vi "Peregrine_write.vi"(0 "Handle in":refnum<visa-resource-name>, 2 "Address":u8, 5 "Key":u32, 7 "Value":i32, 11 "error":errorcluster) -> (4 "Handle out":refnum<visa-resource-name>, 6 "Key response":u32, 8 "Value response":i32, 15 "error out":errorcluster)   [LabVIEW 2019]
panel:
  out "Command":i32
  out "Address response":u8
  # "Inputs"
  # "Response message"
  # "Output"
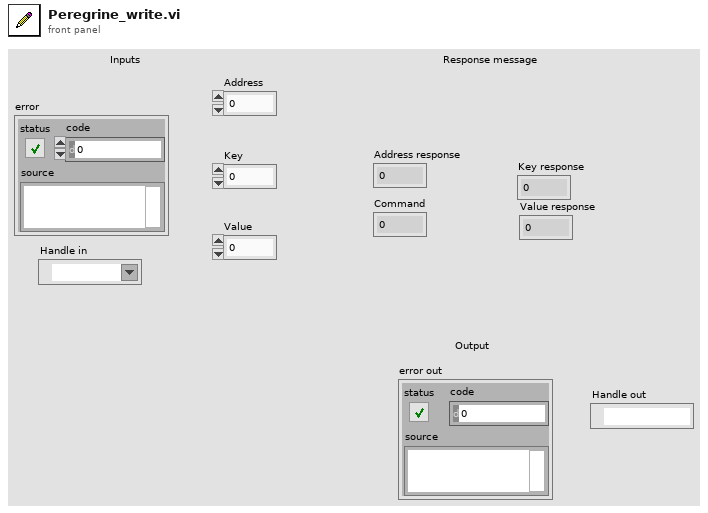
[diagram p1: front panel]
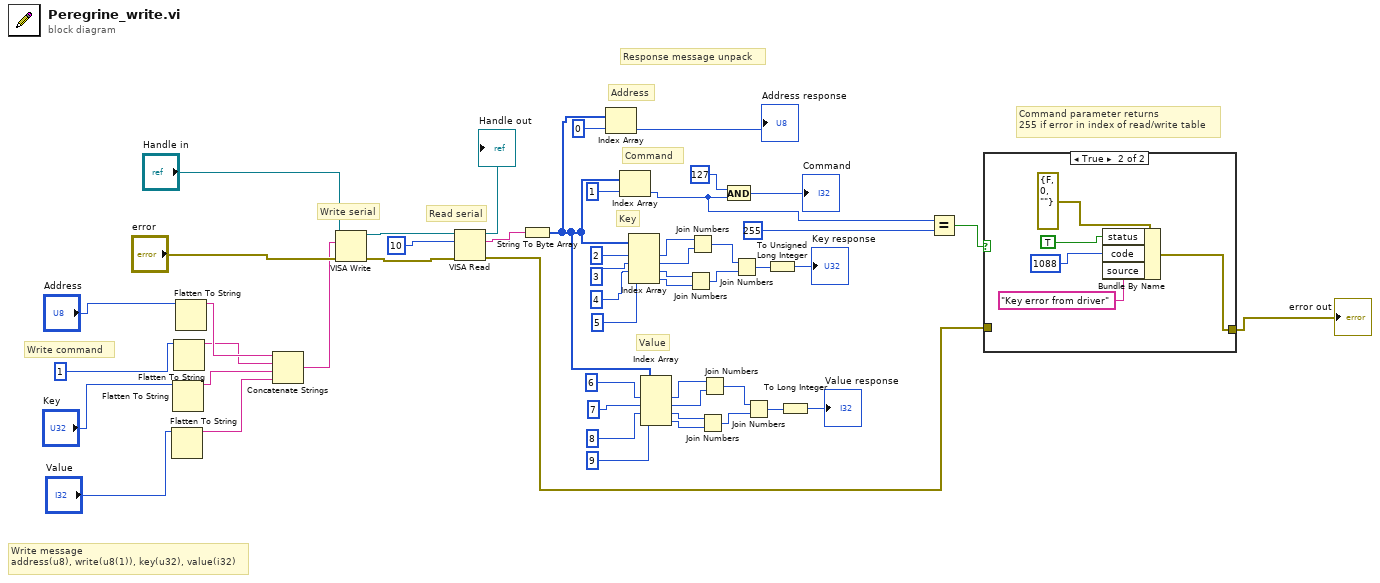
[diagram p0: block diagram]
diagram:
  # "Command parameter returns\n255 if error in index of read/write table"
  # "Value"
  # "Response message unpack"
  # "Write command"
  # "Command"
  # "Address"
  # "Key"
  # "Read serial"
  # "Write serial"
  # "Write message\naddress(u8), write(u8(1)), key(u32), value(i32)"
  n1 = Flatten To String(anything="Value") -> (data string=w24:string)  [unwired: 3 in, 2 out]
  n2 = Flatten To String(anything="Key") -> (data string=w25:string)  [unwired: 3 in, 2 out]
  n3 = Flatten To String(anything=u8 1) -> (data string=w26:string)  [unwired: 3 in, 2 out]
  n4 = Flatten To String(anything="Address") -> (data string=w28:string)  [unwired: 3 in, 2 out]
  n5 = Concatenate Strings(w28, w26, w25, w24) -> (w23:string)
  n6 = VISA Write(VISA resource name="Handle in", write buffer=w23, error in (no error)="error") -> (VISA resource name out=w51:refnum<visa-resource-name>, error out=w30:errorcluster)  [unwired: 1 out]
  n7 = VISA Read(VISA resource name=w51, byte count=10, error in (no error)=w30) -> (VISA resource name out=→"Handle out":refnum<visa-resource-name>, read buffer=w49:string, error out=w3:errorcluster)  [unwired: 1 out]
  n8 = String To Byte Array(string=w49) -> (unsigned byte array=w13:u8[])
  n9 = Index Array(array=w13, index=0) -> (element=→"Address response":u8)
  n10 = Index Array(array=w13, index=1) -> (element=w1:u8)
  n11 = Index Array(array=w13, index #1=2, index #2=3, index #3=4, index #4=5) -> (element #1=w42:u8, element #2=w41:u8, element #3=w40:u8, element #4=w39:u8)
  n12 = Index Array(array=w13, index #1=6, index #2=7, index #3=8, index #4=9) -> (element #1=w20:u8, element #2=w19:u8, element #3=w18:u8, element #4=w17:u8)
  n13 = Join Numbers(hi=w40, lo=w39) -> ((hi.lo)=w38:u16)
  n14 = Join Numbers(hi=w42, lo=w41) -> ((hi.lo)=w37:u16)
  n15 = Join Numbers(hi=w18, lo=w17) -> ((hi.lo)=w16:u16)
  n16 = Join Numbers(hi=w20, lo=w19) -> ((hi.lo)=w15:u16)
  n17 = And(x=127, y=w1) -> (x .and. y?=→"Command":i32)
  n18 = Join Numbers(hi=w37, lo=w38) -> ((hi.lo)=w8:u32)
  n19 = Join Numbers(hi=w15, lo=w16) -> ((hi.lo)=w9:u32)
  n20 = To Unsigned Long Integer(number=w8) -> (unsigned 32bit integer=→"Key response":u32)
  n21 = To Long Integer(number=w9) -> (32bit integer=→"Value response":i32)
  n22 = Equal?(x=w1, y=255) -> (x = y?=w5:bool)
  n23 = case shown="True" w5 {
    tunnel: [w52 w54] -> w4
    tunnel: w3 -> [w52 _]
    frame False {
    }
    frame True {
      n24 = Bundle By Name(cluster=errorcluster {"status"=FALSE, "code"=0, "source"=""} ("error constant"), "status"=TRUE, "code"=1088, "source"="Key error from driver") -> (w54:errorcluster)
    }
  }
  "error out" <- w4
